vi "MD5 Continous Digest.vi"(8 "error in (no error)":errorcluster, 9 "Finish?":bool, 10 "ReInit?":bool, 11 "String":string) -> (0 "error out (pass through)":errorcluster, 3 "MD5 Message Digest":string)   [LabVIEW 2009]
doc: "Implements the MD5 algorithm to produce a 128-bit hash condensed representation of a message or a data file."
panel:
  # "[OpenG VI Tags] ***Do Not Remove***"
  # "MD5 Message Digest.vi\n\nImplements the MD5 algorithm to produce a 128-bit hash condensed representation of a message or a data file. Derived from the RSA Data Security, Inc. MD5 Message-Digest Algorithm\n\nPlease visit http://www.OpenG.org to learn about the\nOpen Source LabVIEW software movement.\n\nNOTICE -- YOU MUST LEAVE THIS NOTICE IN PLACE.  PER THE TERMS OF THE LICENSE BELOW, YOU MAY SUBLICENSE THIS SOFTWARE \nIN ANY WAY THAT DOES NOT CONFLICT WITH THIS LICENSE.\n\n### BSD License (http://www.opensource.org/licenses/bsd-license.php) Begin ###\n \nCopyright (c) 2004, Enrique Vargas <vargas@visecurity.com>\n\nAll rights reserved.\n\nRedistribution and use in source and binary forms, with or without modification, are permitted provided that the following conditions are met:\n\n    * Redistributions of source code must retain the above copyright notice, this list of conditions and the following disclaimer.\n    * Redistributions in binary form must reproduce the above copyright notice, this list of conditions and the following disclaimer in the \n       documentation and/or other materials provided with the distribution.\n    * Neither the name of SciWare, James Kring, Inc., nor the names of its contributors may be used to endorse or promote products derived \n       from this software without specific prior written permission.\n\nTHIS SOFTWARE IS PROVIDED BY THE COPYRIGHT HOLDERS AND CONTRIBUTORS \"AS IS\" AND ANY EXPRESS OR IMPLIED WARRANTIES, \nINCLUDING, BUT NOT LIMITED TO, THE IMPLIED WARRANTIES OF MERCHANTABILITY AND FITNESS FOR A PARTICULAR PURPOSE ARE \nDISCLAIMED. IN NO EVENT SHALL THE COPYRIGHT OWNER OR CONTRIBUTORS BE LIABLE FOR ANY DIRECT, INDIRECT, INCIDENTAL,\n SPECIAL, EXEMPLARY, OR CONSEQUENTIAL DAMAGES (INCLUDING, BUT NOT LIMITED TO, PROCUREMENT OF SUBSTITUTE GOODS OR \nSERVICES; LOSS OF USE, DATA, OR PROFITS; OR BUSINESS INTERRUPTION) HOWEVER CAUSED AND ON ANY THEORY OF LIABILITY, \nWHETHER IN CONTRACT, STRICT LIABILITY, OR TORT (INCLUDING NEGLIGENCE OR OTHERWISE) ARISING IN ANY WAY OUT OF THE USE \nOF THIS SOFTWARE, EVEN IF ADVISED OF THE POSSIBILITY OF SUCH DAMAGE.\n\n### BSD License End ###"
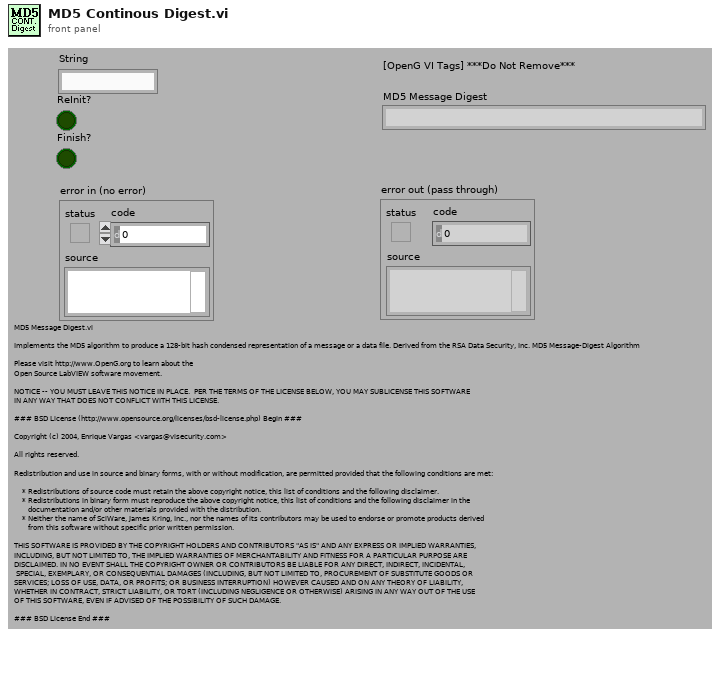
[diagram p1: front panel]
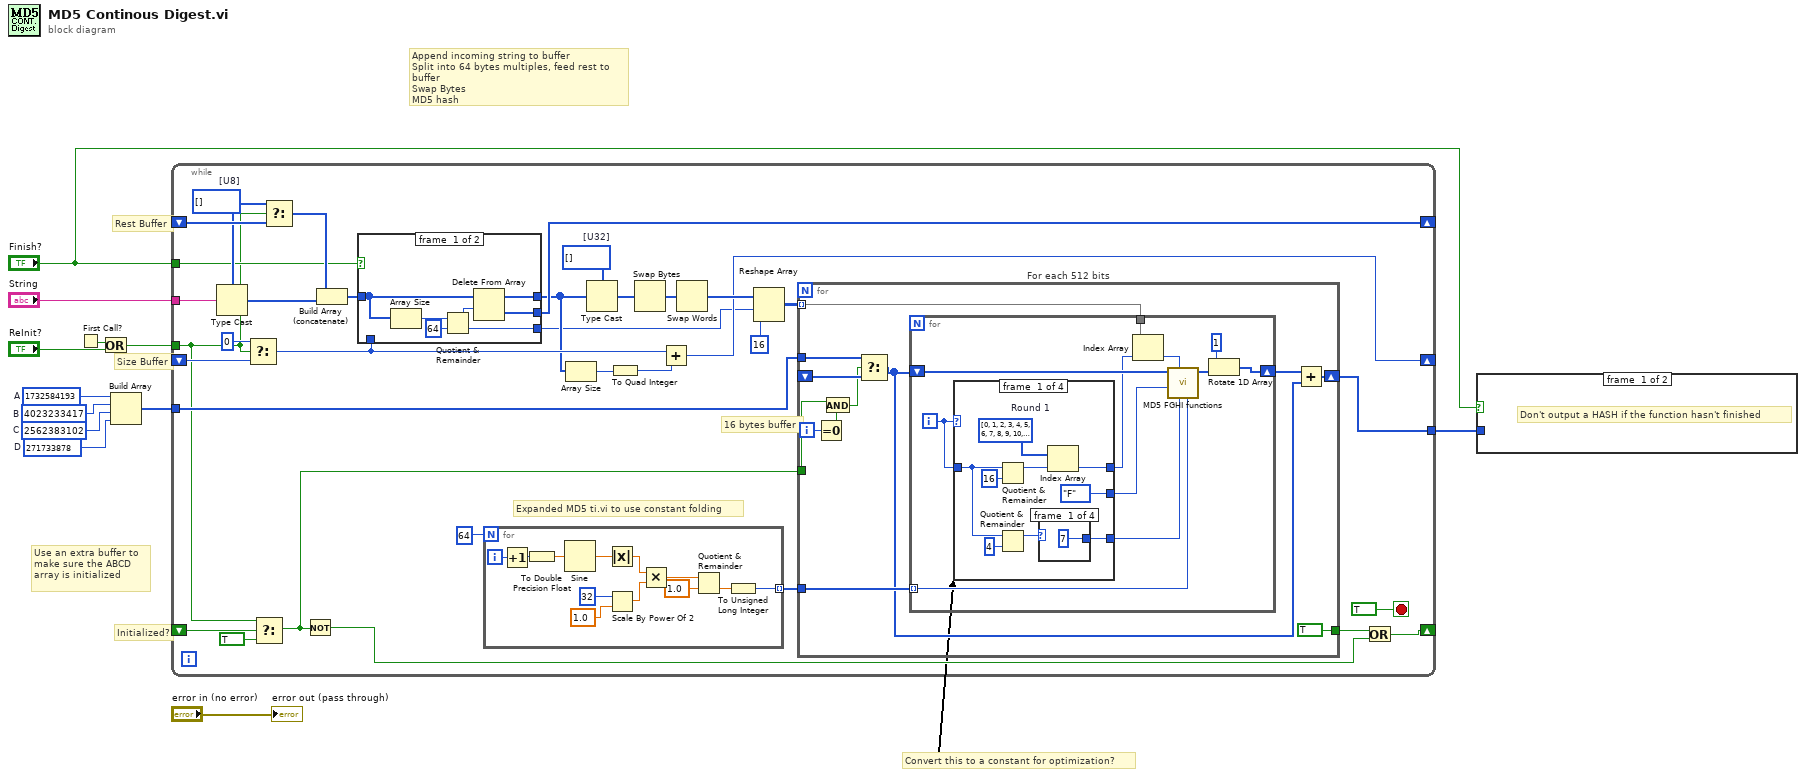
[diagram p0: block diagram]
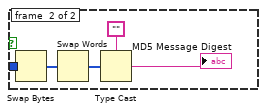
[diagram p2: hidden frame]
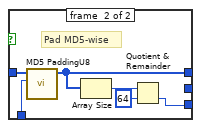
[diagram p3: hidden frame]
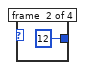
[diagram p4: hidden frame]
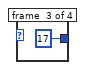
[diagram p5: hidden frame]
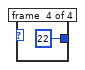
[diagram p6: hidden frame]
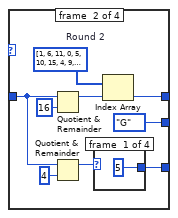
[diagram p7: hidden frame]
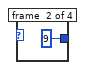
[diagram p8: hidden frame]
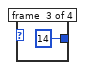
[diagram p9: hidden frame]
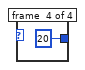
[diagram p10: hidden frame]
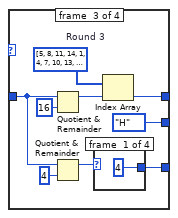
[diagram p11: hidden frame]
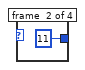
[diagram p12: hidden frame]
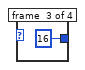
[diagram p13: hidden frame]
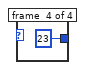
[diagram p14: hidden frame]
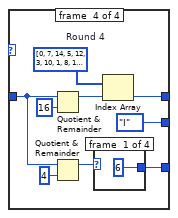
[diagram p15: hidden frame]
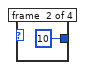
[diagram p16: hidden frame]
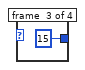
[diagram p17: hidden frame]
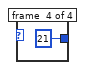
[diagram p18: hidden frame]
diagram:
  w2 = u32 1732584193  # A
  w3 = u32 4023233417  # B
  w4 = u32 2562383102  # C
  w5 = u32 271733878  # D
  # "Convert this to a constant for optimization?"
  # "Initialized?"
  # "Use an extra buffer to \nmake sure the ABCD\narray is initialized"
  # "Append incoming string to buffer\nSplit into 64 bytes multiples, feed rest to buffer\nSwap Bytes\nMD5 hash"
  # "Rest Buffer"
  # "Size Buffer"
  n1 = First Call?() -> (First Call?: T/F=w11:bool)
  n2 = Or(x=w11, y="ReInit?") -> (x .or. y?=w10:bool)
  n3 = Build Array(w2, w3, w4, w5) -> (w1:u32[])
  n4 = while {
    tunnel: "String" -> [w33]
    shift-right: [w23] -> _
    shift-left: _ -> [w42]
    tunnel: w10 -> [w15]
    shift-right: [w34] -> _
    shift-left: _ -> [w41]
    tunnel: "Finish?" -> [w31]
    tunnel: [w21] -> w8
    shift-right: [w19] -> _
    shift-left: _ -> [w17]
    tunnel: w1 -> [w18]
    stop <- TRUE stop-if-true
    w29 = u32[] []  # [U32]
    w38 = u8[] []  # [U8]
    # "Expanded MD5 ti.vi to use constant folding"
    # "16 bytes buffer"
    n5 = Type Cast(type=w38, x=w33) -> (*(type *) &x=w32:u8[])
    n6 = Select(t=i64 0, s=w15, f=w42) -> (s? t:f=w30:i64)
    n7 = Select(t=w15, s=w17, f=TRUE ("t")) -> (s? t:f=w14:bool)
    n8 = Select(t=w38, s=w15, f=w41) -> (s? t:f=w37:u8[])
    n9 = Not(x=w14) -> (.not. x?=w13:bool)
    n10 = Build Array (concatenate)(w37, w32) -> (w36:u8[])
    n11 = case shown="True" w31 {
      tunnel: w36 -> [w53 w56]
      tunnel: [w52 _] -> w34
      tunnel: [w48 w57] -> w22
      tunnel: [w47 w54] -> w27
      tunnel: w30 -> [_ w55]
      frame #0 {
        n12 = Array Size(array=w53) -> (size(s)=w51:i32)
        n13 = Quotient & Remainder(x=w51, y=64) -> (x-y*floor(x/y)=w49:i32, floor(x/y)=w48:i32)
        n14 = Delete From Array(array=w53, length=w49) -> (deleted portion=w52:u8[], array with subset deleted=w47:u8[])  [unwired: 1 in]
      }
      frame #1 {
        # "Pad MD5-wise"
        n15 = call "MD5 PaddingU8.vi"("Pre Buffer Size"=w55, "Current Buffer"=w56) -> ("MD5 Padded Buffer"=w54:u8[])  [unwired: 9 in]
        n16 = Array Size(array=w54) -> (size(s)=w59:i32)
        n17 = Quotient & Remainder(x=w59, y=64) -> (floor(x/y)=w57:i32)  [unwired: 1 out]
      }
    }
    n18 = for {
      N: 64 -> [_]
      tunnel: [w60] -> w45 mode=indexing
      i -> [w71]
      n19 = Increment(x=w71) -> (x+1=w61:i32)
      n20 = To Double Precision Float(number=w61) -> (double precision float=w69:dbl)
      n21 = Sine(x=w69) -> (sin(x)=w70:dbl)
      n22 = Absolute Value(x=w70) -> (abs(x)=w66:dbl)
      n23 = Scale By Power Of 2(n=32, x=1.0) -> (x*2^n=w65:dbl)
      n24 = Multiply(x=w66, y=w65) -> (x*y=w64:dbl)
      n25 = Quotient & Remainder(x=w64, y=1.0) -> (floor(x/y)=w62:dbl)  [unwired: 1 out]
      n26 = To Unsigned Long Integer(number=w62) -> (unsigned 32bit integer=w60:u32)
    }
    n27 = Array Size(array=w27) -> (size(s)=w40:i32)
    n28 = Type Cast(type=w29, x=w27) -> (*(type *) &x=w25:u32[])
    n29 = To Quad Integer(1:w40) -> (0:w39:i64)
    n30 = Swap Bytes(anything=w25) -> (byte swapped=w26:u32[])
    n31 = Add(x=w30, y=w39) -> (x+y=w23:i64)
    n32 = Swap Words(1:w26) -> (0:w24:u32[])
    n33 = Reshape Array(w24, w22, 16 ("dimension size")) -> (w28:u32[][])
    n34 = for "For each 512 bits" {
      shift-right: [w83] -> w21
      shift-left: _ -> [w78]
      tunnel: w28 -> [w81] mode=indexing
      tunnel: w45 -> [w80]
      tunnel: w18 -> [w79]
      tunnel: [TRUE] -> w20
      tunnel: w14 -> [w72]
      i -> [w76]
      n35 = Equal To 0?(x=w76) -> (x = 0?=w75:bool)
      n36 = And(x=w72, y=w75) -> (x .and. y?=w74:bool)
      n37 = Select(t=w79, s=w74, f=w78) -> (s? t:f=w77:u32[])
      n38 = for {
        tunnel: w81 -> [w88]
        shift-right: [w93] -> w82
        shift-left: w77 -> [w91]
        tunnel: w80 -> [w84] mode=indexing
        i -> [w92]
        n39 = case shown="16..31" w92 {
          tunnel: w92 -> [w100 w114 w127 w140]
          tunnel: [enum16{"F", "G", "H", "I"}."F" ("Operator function") enum16{"F", "G", "H", "I"}."G" ("Operator function") enum16{"F", "G", "H", "I"}."H" ("Operator function") enum16{"F", "G", "H", "I"}."I" ("Operator function")] -> w86
          tunnel: [w96 w109 w122 w135] -> w85
          tunnel: [w95 w108 w121 w134] -> w89
          frame #0 {
            w99 = i32[] [0, 1, 2, 3, 4, 5, 6, 7, 8, 9, 10, 11, 12, 13, 14, 15]  # Round 1
            n40 = Quotient & Remainder(x=w100, y=16) -> (x-y*floor(x/y)=w98:i32)  [unwired: 1 out]
            n41 = Quotient & Remainder(x=w100, y=4) -> (x-y*floor(x/y)=w102:i32)  [unwired: 1 out]
            n42 = case shown="0, Default" w102 {
              tunnel: [7 ("s") 12 ("s") 17 ("s") 22 ("s")] -> w96
              frame #0 {
              }
              frame #1 {
              }
              frame #2 {
              }
              frame #3 {
              }
            }
            n43 = Index Array(array=w99, index=w98) -> (element=w95:i32)
          }
          frame #1 {
            w112 = i32[] [1, 6, 11, 0, 5, 10, 15, 4, 9, 14, 3, 8, 13, 2, 7, 12]  # Round 2
            n44 = Quotient & Remainder(x=w114, y=16) -> (x-y*floor(x/y)=w113:i32)  [unwired: 1 out]
            n45 = Quotient & Remainder(x=w114, y=4) -> (x-y*floor(x/y)=w111:i32)  [unwired: 1 out]
            n46 = case shown="0, Default" w111 {
              tunnel: [5 ("s") 9 ("s") 14 ("s") 20 ("s")] -> w109
              frame #0 {
              }
              frame #1 {
              }
              frame #2 {
              }
              frame #3 {
              }
            }
            n47 = Index Array(array=w112, index=w113) -> (element=w108:i32)
          }
          frame #2 {
            w125 = i32[] [5, 8, 11, 14, 1, 4, 7, 10, 13, 0, 3, 6, 9, 12, 15, 2]  # Round 3
            n48 = Quotient & Remainder(x=w127, y=16) -> (x-y*floor(x/y)=w126:i32)  [unwired: 1 out]
            n49 = Quotient & Remainder(x=w127, y=4) -> (x-y*floor(x/y)=w124:i32)  [unwired: 1 out]
            n50 = case shown="0, Default" w124 {
              tunnel: [4 ("s") 11 ("s") 16 ("s") 23 ("s")] -> w122
              frame #0 {
              }
              frame #1 {
              }
              frame #2 {
              }
              frame #3 {
              }
            }
            n51 = Index Array(array=w125, index=w126) -> (element=w121:i32)
          }
          frame #3 {
            w138 = i32[] [0, 7, 14, 5, 12, 3, 10, 1, 8, 15, 6, 13, 4, 11, 2, 9]  # Round 4
            n52 = Quotient & Remainder(x=w140, y=16) -> (x-y*floor(x/y)=w139:i32)  [unwired: 1 out]
            n53 = Quotient & Remainder(x=w140, y=4) -> (x-y*floor(x/y)=w137:i32)  [unwired: 1 out]
            n54 = case shown="0, Default" w137 {
              tunnel: [6 ("s") 10 ("s") 15 ("s") 21 ("s")] -> w135
              frame #0 {
              }
              frame #1 {
              }
              frame #2 {
              }
              frame #3 {
              }
            }
            n55 = Index Array(array=w138, index=w139) -> (element=w134:i32)
          }
        }
        n56 = Index Array(array=w88, index=w89) -> (element=w87:u32)
        n57 = call "MD5 FGHI functions.vi"("ti"=w84, "s"=w85, "Mj"=w87, "Operator function"=w86, "Chaining Variables"=w91) -> ("Resulting Chaining Variables"=w90:u32[])  [unwired: 6 in]
        n58 = Rotate 1D Array(1:w90, 2:1 ("n")) -> (0:w93:u32[])
      }
      n59 = Add(x=w82, y=w77) -> (x+y=w83:u32[])
    }
    n60 = Or(x=w20, y=w13) -> (x .or. y?=w19:bool)
  }
  n61 = case shown="True" "Finish?" {
    tunnel: w8 -> [_ w147]
    frame #0 {
      # "Don't output a HASH if the function hasn't finished"
    }
    frame #1 {
      n62 = Swap Bytes(anything=w147) -> (byte swapped=w150:u32[])
      n63 = Swap Words(1:w150) -> (0:w151:u32[])
      n64 = Type Cast(type="", x=w151) -> (*(type *) &x=→"MD5 Message Digest":string)
    }
  }
  "error out (pass through)" <- "error in (no error)"
